vi "FindChildProjItem.vi"(10 "Level":string[](array[string]), 11 "ProjectItem in":refnum<vi>) -> (2 "Found?":bool, 3 "Found or Orig":refnum<vi>)   [LabVIEW 2024, in "AddNewEvent.lvlib"]
uses:
  AddNewEvent.lvlib
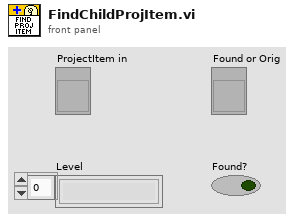
[diagram p1: front panel]
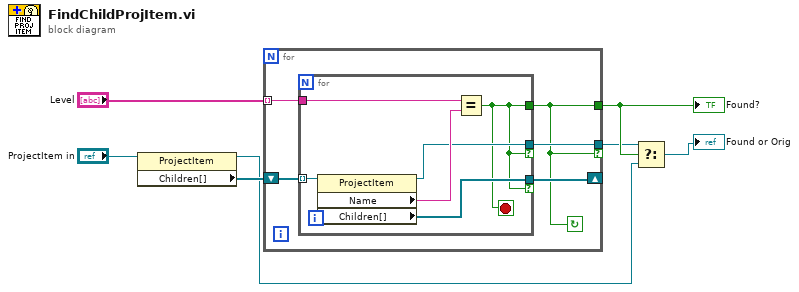
[diagram p0: block diagram]
diagram:
  n1 = property class="ProjectItem"(reference="ProjectItem in") -> (reference out=w2:refnum<vi>, "Children[]"=w5:refnum<vi>[])  [unwired: 1 in, 1 out]
  n2 = for {
    tunnel: "Level" -> [w11] mode=indexing
    tunnel: [w8] -> w4
    shift-right: [w10] -> _
    shift-left: w5 -> [w12]
    tunnel: [w9] -> w3 if=w8
    stop <- w8 continue-if-true
    n3 = for {
      tunnel: w12 -> [w18] mode=indexing
      tunnel: w11 -> [w17]
      tunnel: [w13] -> w8
      tunnel: [w15] -> w10 if=w13
      tunnel: [w14] -> w9 if=w13
      stop <- w13 stop-if-true
      n4 = property class="ProjectItem"(reference=w18) -> (reference out=w14:refnum<vi>, "Name"=w16:string, "Children[]"=w15:refnum<vi>[])  [unwired: 1 in, 1 out]
      n5 = Equal?(x=w17, y=w16) -> (x = y?=w13:bool)
    }
  }
  "Found?" <- w4
  n6 = Select(t=w3, s=w4, f=w2) -> (s? t:f=→"Found or Orig":refnum<vi>)
